vi "Read Int from ROS.vi"() -> ()   [LabVIEW 2018]
uses:
  <vilib>/RTI DDS Toolkit/Types/RTI DDS Advanced Reader Configuration.ctl
  <vilib>/RTI DDS Toolkit/VIs/AdvancedCreateReader_NumI32.vi
  <vilib>/RTI DDS Toolkit/VIs/Read_NumI32.vi
  <vilib>/RTI DDS Toolkit/Library/LVDDS_library.lvlib
panel:
  out "Int from ros":i32
  in  "stop":bool
  in  "error in (no error)":errorcluster
  in  "Advanced Reader Configuration":T1={"typeName"="std_msgs::msg::dds_::Int32_", "keyName"="", "domainParticipantQoSProfile"="", "dataReaderQoSProfile"="", "forceArrayMapping?"=FALSE, "forceExclusiveReader?"=FALSE, "forceRead? (only ExclusiveReader)"=FALSE, "forceUnboundedString?"=FALSE}
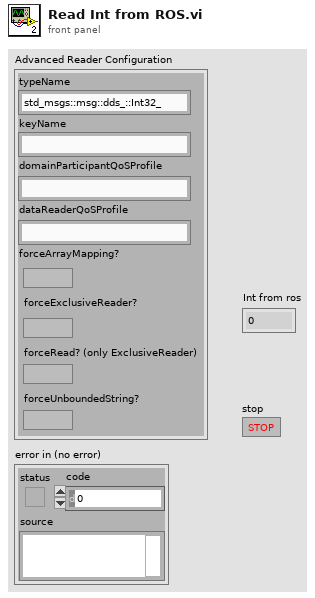
[diagram p1: front panel]
types:
  T1 = typedef "LVDDS_library.lvlib/RTI DDS Advanced Reader Configuration.ctl" = cluster{"typeName":string, "keyName":string, "domainParticipantQoSProfile":string, "dataReaderQoSProfile":string, "forceArrayMapping?":bool, "forceExclusiveReader?":bool, "forceRead? (only ExclusiveReader)":bool, "forceUnboundedString?":bool}
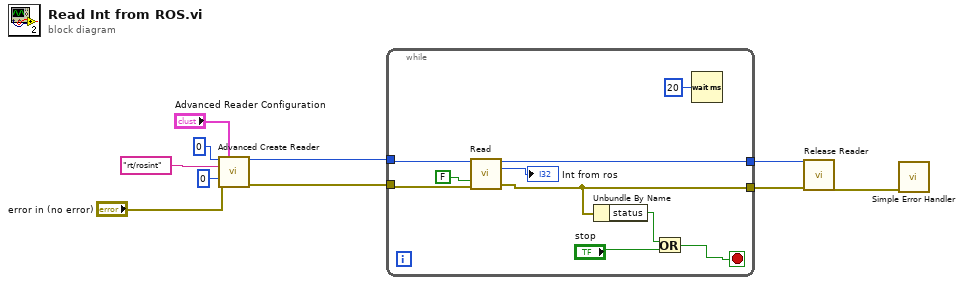
[diagram p0: block diagram]
diagram:
  n1 = call-poly <vilib>:"Advanced Create Reader.vi"("Domain Id"=u32 0 ("Domain id"), "Advanced Reader Configuration"="Advanced Reader Configuration", "Topic Name"="rt/rosint", "Data Type"=0, "error in (no error)"="error in (no error)") -> ("DDS Object Ref"=w5:u64, "error out"=w4:errorcluster)  [unwired: 9 in]
  n2 = while {
    tunnel: w5 -> [w20]
    tunnel: w4 -> [w19]
    tunnel: [w16] -> w3
    tunnel: [w15] -> w2
    stop <- w12 stop-if-true
    n3 = call-poly <vilib>:"Read.vi"("DDS Object Ref in"=w20, "Only New Samples"=FALSE, "error in (no error)"=w19) -> ("DDS Object Ref out"=w16:u64, "Data"=→"Int from ros":i32, "error out"=w15:errorcluster)  [unwired: 8 in, 2 out]
    n4 = Unbundle By Name(w15) -> ("status"=w14:bool)
    n5 = Or(x=w14, y="stop") -> (x .or. y?=w12:bool)
    n6 = Wait (ms)(milliseconds to wait=u32 20) -> ()  [unwired: 1 out]
  }
  n7 = call <vilib>:"Release Reader.vi"("error in (no error)"=w2, "DDS Object Ref"=w3) -> ("error out"=w1:errorcluster)  [unwired: 9 in]
  n8 = call <vilib>:"Simple Error Handler.vi"("error in (no error)"=w1) -> ()  [unwired: 4 in, 5 out]
